vi "Process.vi"(8 "error in":errorcluster, 11 "Inst.SPC":refnum<class "Inst.SPC.lvclass">) -> (0 "error out":errorcluster, 3 "Inst.SPC out":refnum<class "Inst.SPC.lvclass">)   [LabVIEW 2019, in "Inst.SPC.lvclass"]
doc: "---------------------------------------------------------------\nJKI State Machine Objects™\nhttp://jki.net/state-machine-objects/\nCopyright (C) 2005-2015, JKI <info@jki.net>\nALL RIGHTS RESERVED"
uses:
  Inst.SPC.lvclass
  C:/Program Files (x86)/National Instruments/LabVIEW 2019/vi.lib/JKI/JKI SMO/SMO/SMO.lvclass
  C:/Program Files (x86)/National Instruments/LabVIEW 2019/user.lib/LevyLab/Instrument Framework/SMOs/Instrument/Instrument.lvclass
  Typedefs/PrivateEvents--Inst.SPC.MessageToProcess.ctl
  <userlib>/LevyLab/Instrument Framework/SMOs/RemoteControl/Typedefs/Message--Cluster.ctl
  <vilib>/JKI/JKI SMO/SMO/SMO.lvclass/SMO.ctl
  Inst.SPC.lvclass/Inst.SPC.ctl
  <vilib>/JKI/JKI SMO/SMO/Private/ReftoDVR--SMO.vi
  <userlib>/LevyLab/Instrument Framework/Instrument Types/VSource/Instrument.VSource.lvclass
  <vilib>/JKI/JKI SMO/SMO/SMO.lvclass
  <userlib>/LevyLab/Instrument Framework/SMOs/Instrument/Instrument.lvclass
  <userlib>/LevyLab/Instrument Framework/SMOs/RemoteControl/RemoteControl.lvclass
  C:/Program Files (x86)/National Instruments/LabVIEW 2019/user.lib/LevyLab/Instrument Framework/Instrument Types/VSource/Instrument.VSource.lvclass
  Typedefs/Inst.SPC.Configuration--Cluster.ctl
panel:
  out "Status":string
  out "State History":string
  # "Instrument.SPC"
  # "SPC"
  # "For instructions on how to use the JKI State Machine Objects, examples and video tutorials, visit:\nhttp://jki.net/state-machine-objects/\n\nJKI State Machine Objects™\nhttp://jki.net/state-machine-objects/\nCopyright (C) 2005-2015, JKI <info@jki.net>\nALL RIGHTS RESERVED"
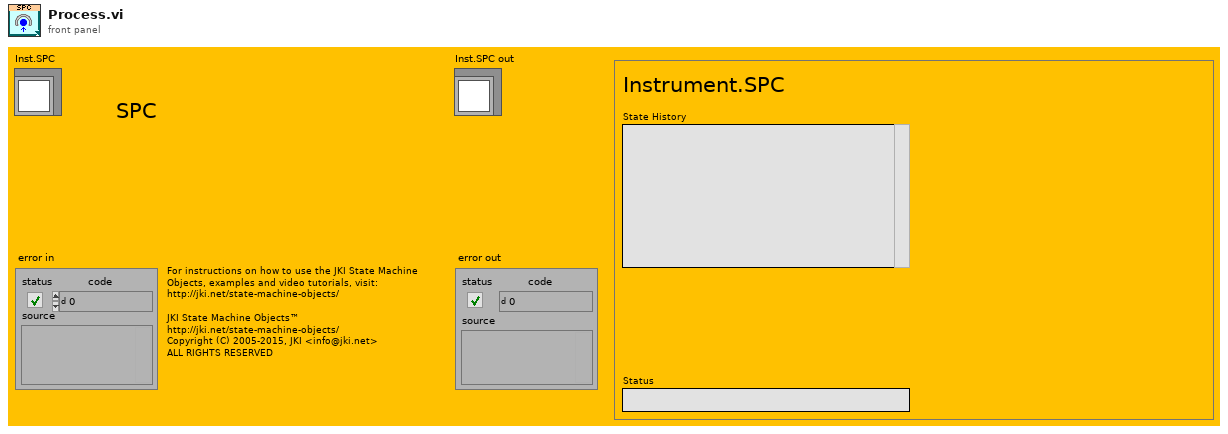
[diagram p1: front panel]
types:
  T1 = enum32{"invalid app kind", "Development System", "Run Time System", "Student Edition", "Embedded LabVIEW", "Evaluation", "Custom"}
  T2 = enum32{"Invalid", "Standard", "Closed", "Hidden", "Minimized", "Maximized"}
  T3 = typedef "Inst.SPC.lvclass/Inst.SPC.Configuration--Cluster.ctl" = cluster{"DCC_DLL":path, "SPC_DLL":path, "DCC_Serials":string[], "SPC_Serials":string[]}
  T4 = typedef "RemoteControl.lvclass/Message--Cluster.ctl" = cluster{"Command":string, "Data":variant, "ID":string}
  T5 = typedef "Inst.SPC.lvclass/PrivateEvents--Inst.SPC.MessageToProcess.ctl" = cluster{"Message":T4}
  T6 = cluster{"Core":cluster{"Current VI Reference":refnum<vi>, "Close Panel on Exit?":bool, "Last Error":cluster{"error":errorcluster, "previous state":string, "remaining states":string}, "Shutdown?":bool}, "SelfRef":refnum<class "Inst.SPC.lvclass">, "Running Step":i32, "sequence":string[], "MessageToProcess":T5}
  T7 = cluster{"Current VI Reference":refnum<vi>, "Close Panel on Exit?":bool, "Last Error":cluster{"error":errorcluster, "previous state":string, "remaining states":string}, "Shutdown?":bool}
  T8 = typedef "SMO.lvclass/Protected Events.ctl" = cluster{"StopProcesses":refnum<user-event>, "AbortProcesses":refnum<user-event>, "Config Changed":refnum<user-event>, "Dependency":refnum<user-event>}
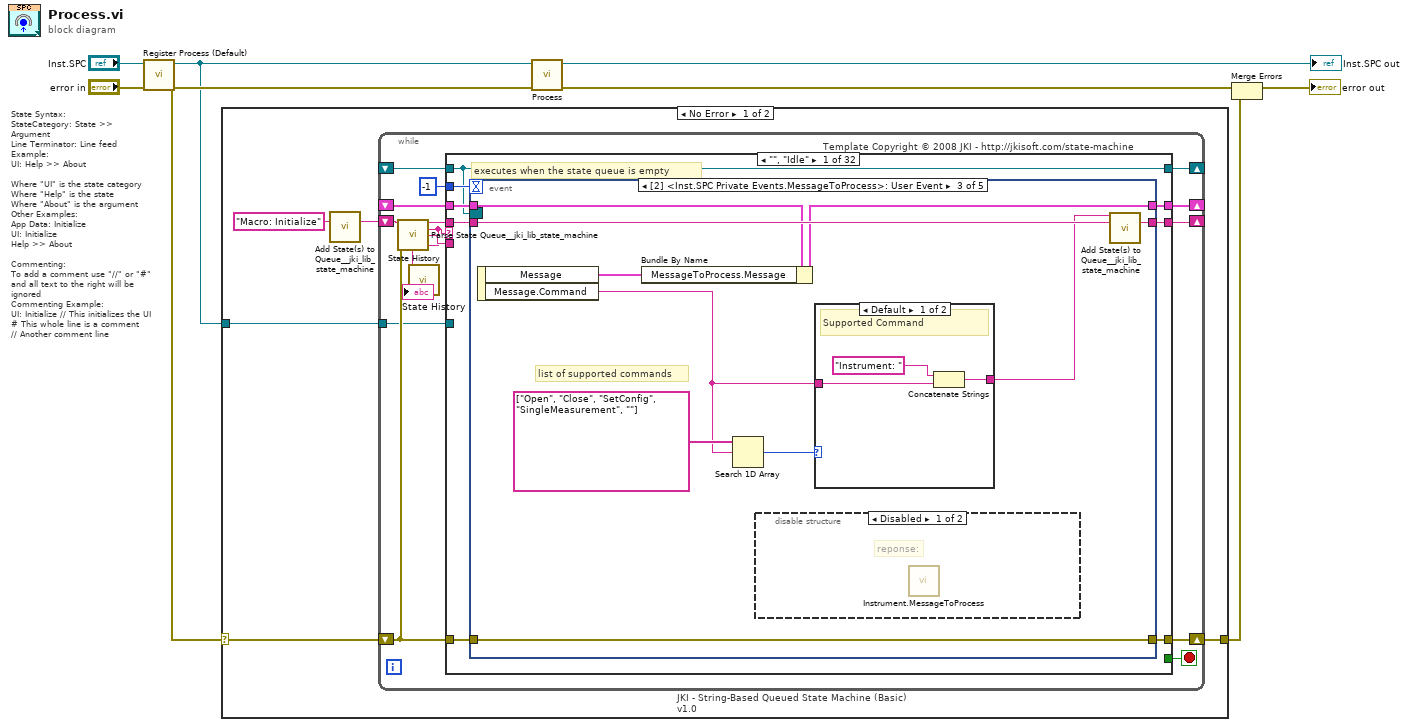
[diagram p0: block diagram]
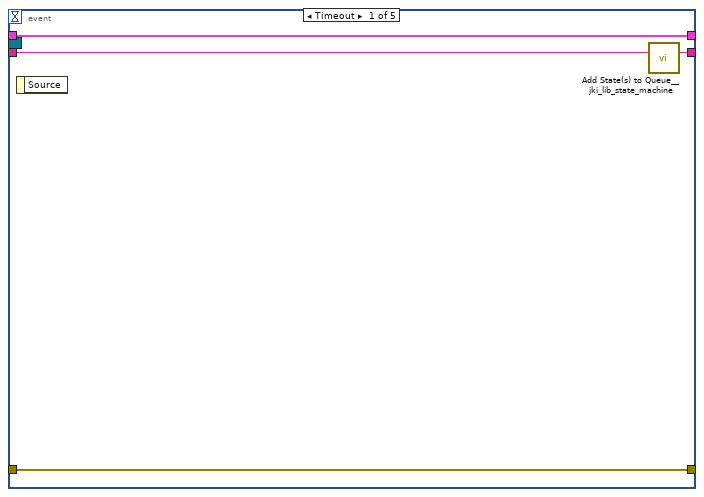
[diagram p2: hidden frame]
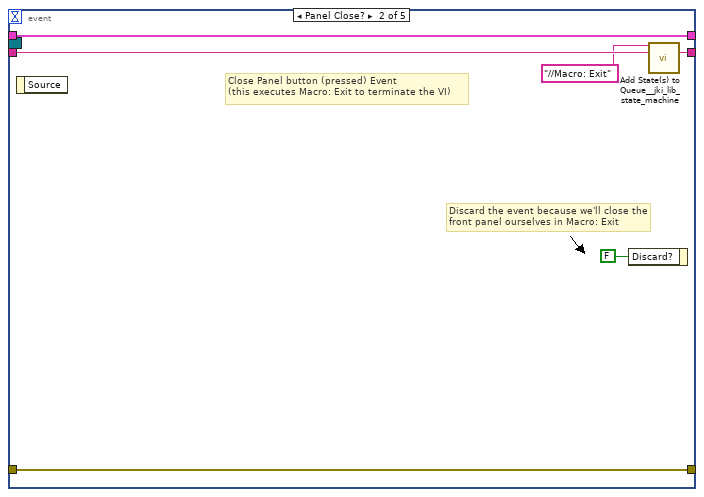
[diagram p3: hidden frame]
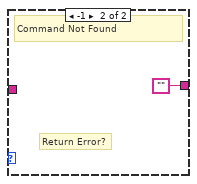
[diagram p5: hidden frame]
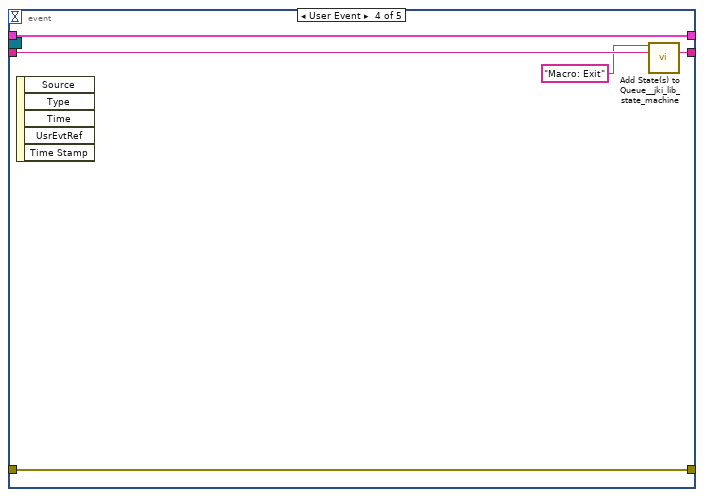
[diagram p6: hidden frame]
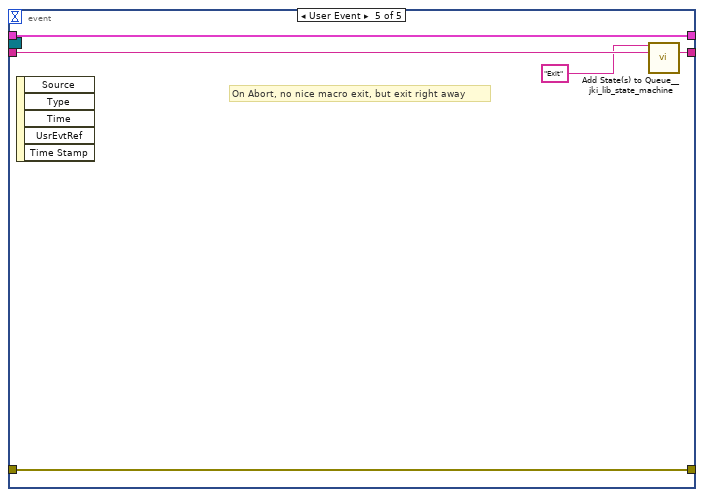
[diagram p7: hidden frame]
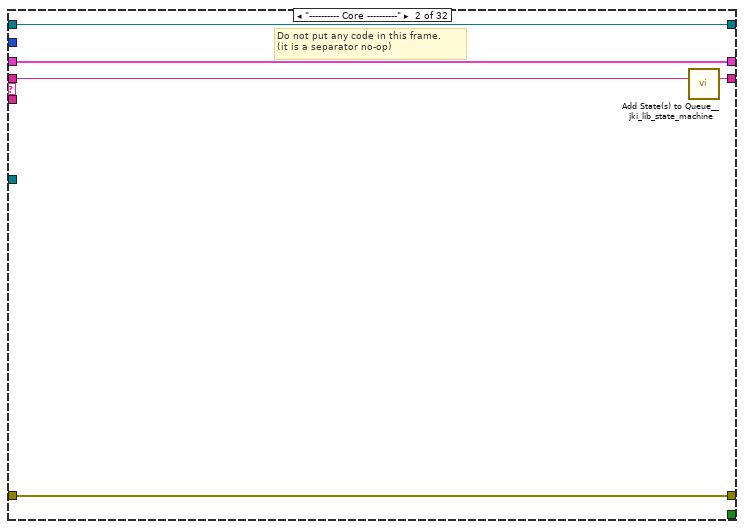
[diagram p8: hidden frame]
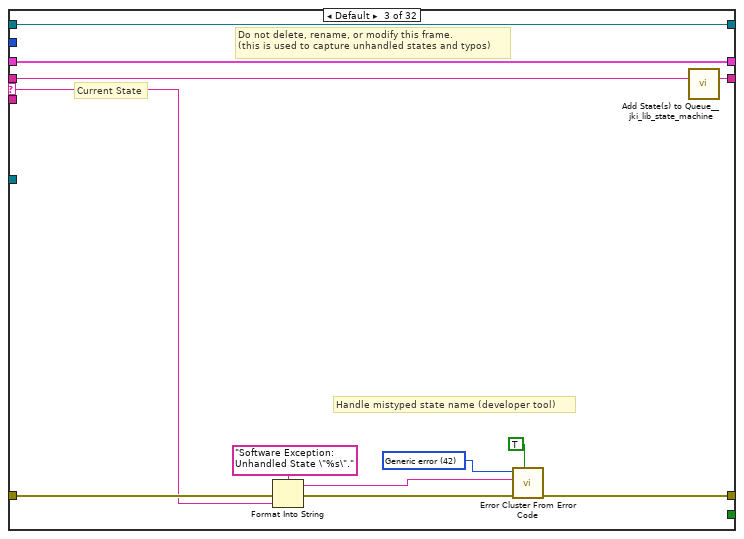
[diagram p9: hidden frame]
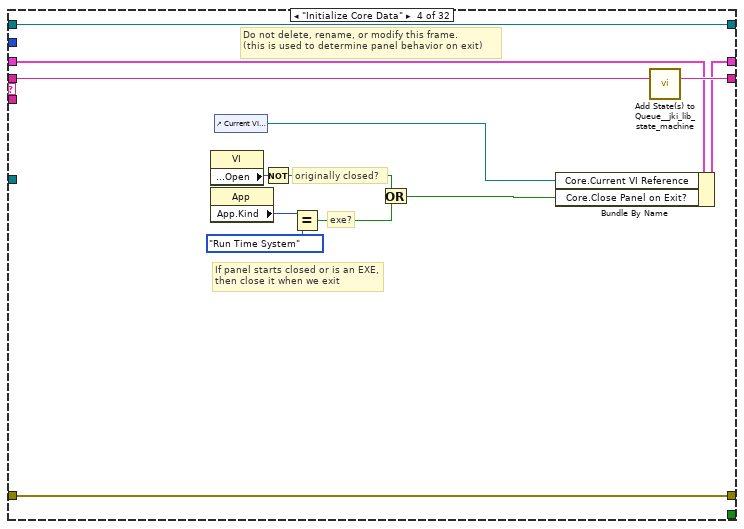
[diagram p10: hidden frame]
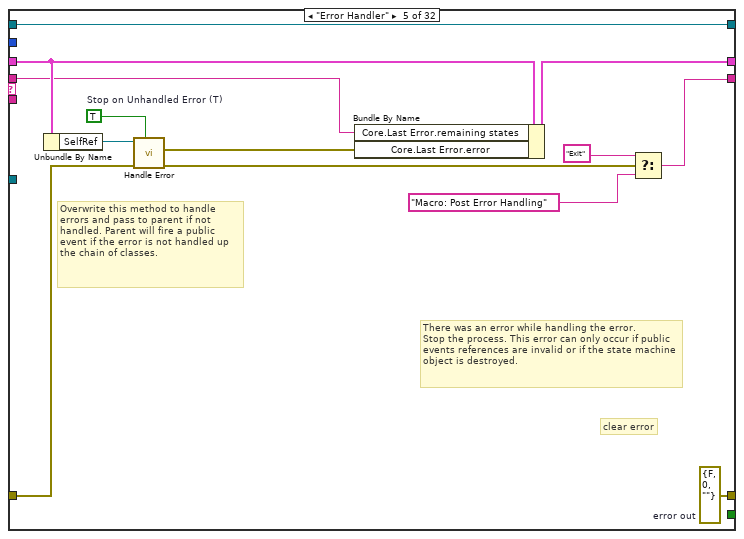
[diagram p11: hidden frame]
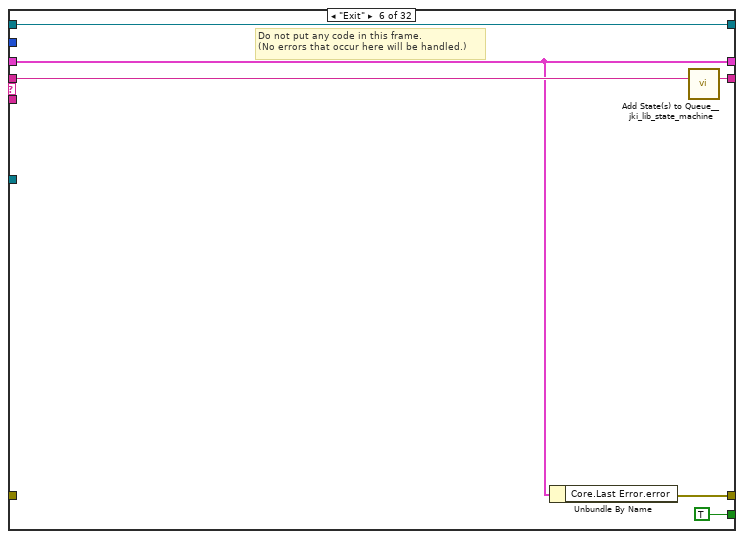
[diagram p12: hidden frame]
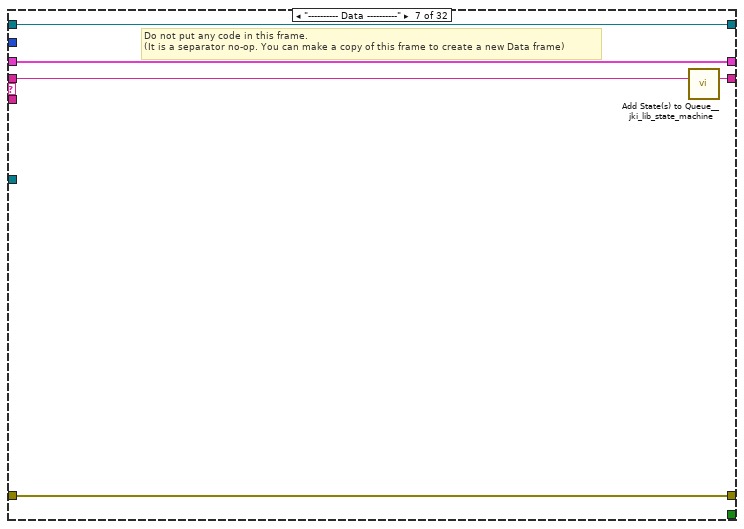
[diagram p13: hidden frame]
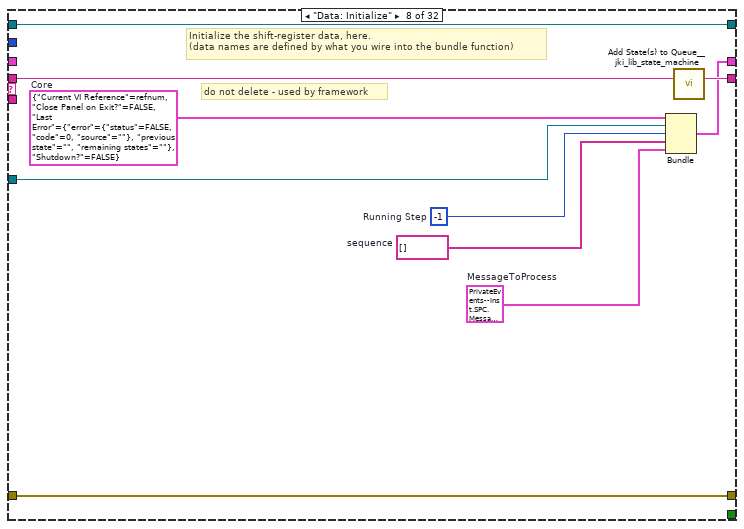
[diagram p14: hidden frame]
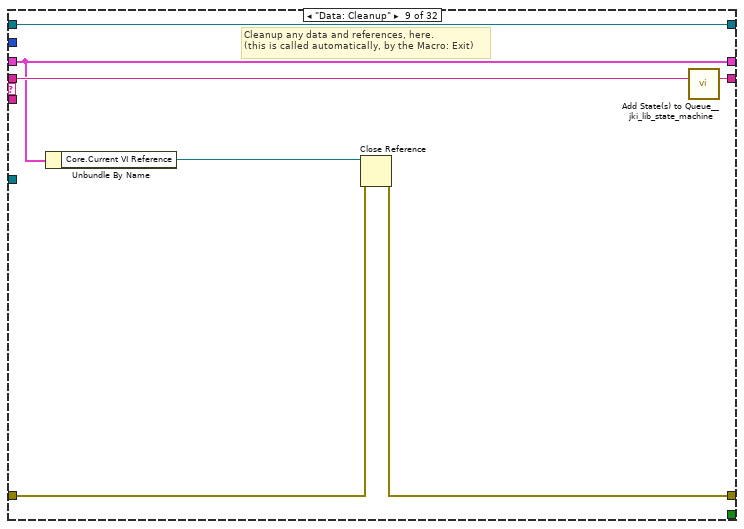
[diagram p15: hidden frame]
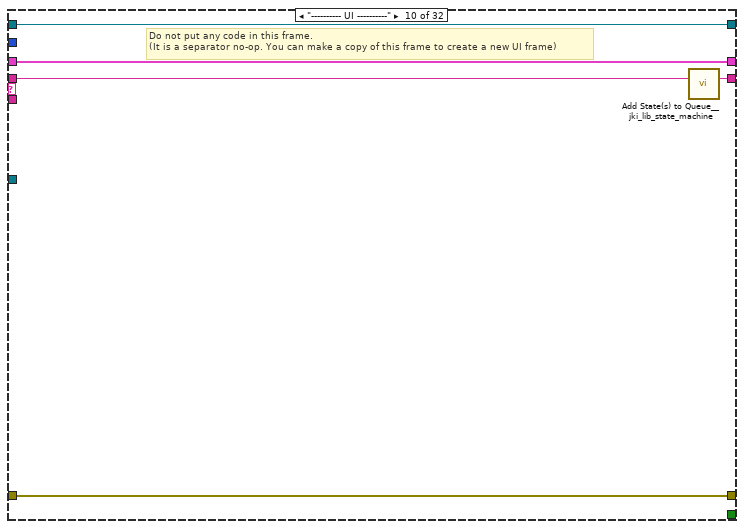
[diagram p16: hidden frame]
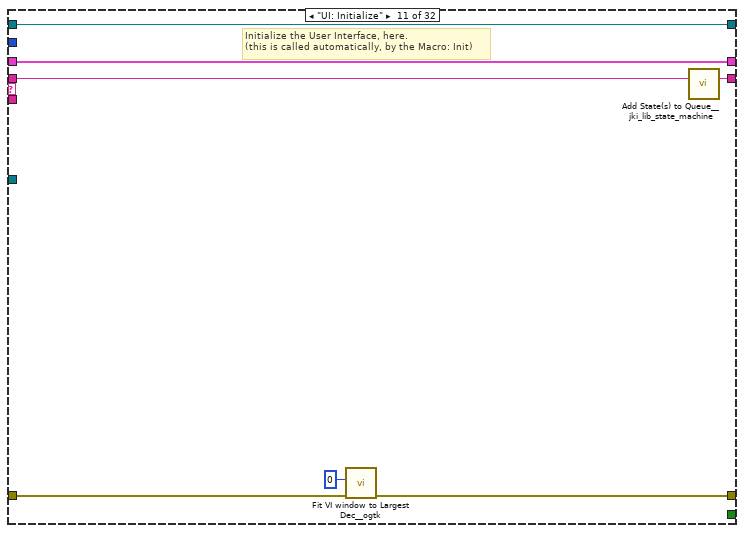
[diagram p17: hidden frame]
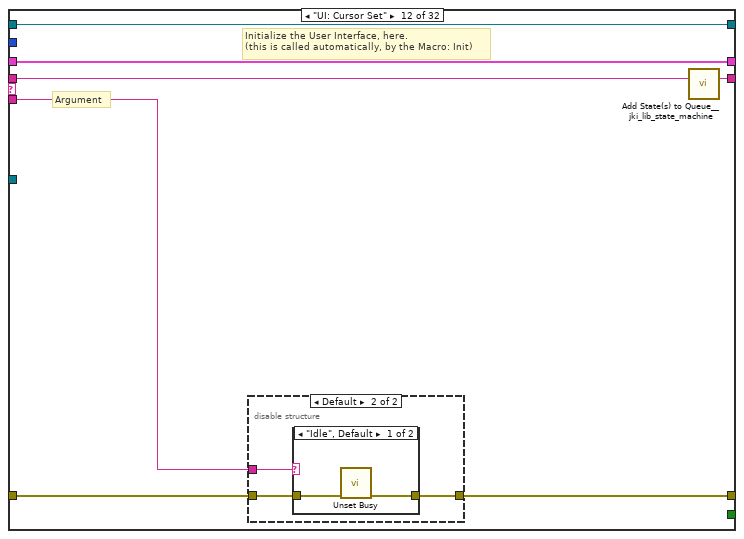
[diagram p18: hidden frame]
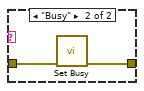
[diagram p20: hidden frame]
diagram:
  # "State Syntax:\nStateCategory: State >> Argument\nLine Terminator: Line feed\nExample:\nUI: Help >> About\n\nWhere \"UI\" is the state category\nWhere \"Help\" is the state\nWhere \"About\" is the argument\nOther Examples:\nApp Data: Initialize\nUI: Initialize\nHelp >> About\n\nCommenting:\nTo add a comment use \"//\" or \"#\" and all text to the right will be ignored\nCommenting Example:\nUI: Initialize // This initializes the UI\n# This whole line is a comment\n// Another comment line"
  n1 = call <vilib>:"Register Process (Default).vi"("error in (no error)"="error in", "SMO"="Inst.SPC") -> ("error out"=w5:errorcluster, "SelfRef"=w4:refnum<class "Inst.SPC.lvclass">)  [unwired: 8 in]
  n2 = case shown="No Error" w5 {
    selector: w5 -> [w10 w422]
    tunnel: w4 -> [w11 _]
    tunnel: [w9 w422] -> w1
    frame No Error {
      n3 = call <vilib>:"Add State(s) to Queue__jki_lib_state_machine.vi"("State(s) in (\"\")"="Macro: Initialize") -> ("States Out"=w13:string)  [unwired: 14 in]
      n4 = while "JKI - String-Based Queued State Machine (Basic) v1.0" {
        shift-right: [w22] -> _
        shift-left: _ -> [w21]
        shift-right: [w25] -> w9
        shift-left: w10 -> [w19]
        shift-right: [w24] -> _
        shift-left: w13 -> [w26]
        tunnel: w11 -> [w18]
        shift-right: [w17] -> _
        shift-left: _ -> [w16]
        stop <- w23 stop-if-true
        # "Template Copyright © 2008 JKI - http://jkisoft.com/state-machine"
        n5 = call <vilib>:"Parse State Queue__jki_lib_state_machine.vi"("State Queue"=w26, "Error In (no error)"=w19) -> ("Remaining States"=w28:string, "Current State"=w15:string, "Arguments"=w27:string)  [unwired: 11 in]
        n6 = call <userlib>:"State History.vi"("Current State"=w15) -> ("History"=→"State History":string)  [unwired: 10 in]
        n7 = case shown="\"\", \"Idle\"" w15 {
          selector: w15 -> [_ _ w77 _ _ _ _ _ _ _ _ _ _ _ _ _ _ _ _ _ _ _ _ _ _ _ _ _ _ _ _ _]
          tunnel: w28 -> [w36 w75 w81 w100 w105 w119 w124 w134 w141 w146 w153 w160 w176 w208 w227 w239 w260 w282 w287 w298 w303 w316 w322 w329 w341 w350 w357 w367 w382 w396 w402 w421]
          tunnel: w27 -> [_ _ _ _ _ _ _ _ _ _ _ w154 w170 _ _ _ _ _ _ _ _ _ _ _ _ _ _ _ _ _ w397 w405]
          tunnel: w21 -> [w34 w72 w79 w91 w109 w115 w121 _ w136 w143 w151 w158 w172 w205 w224 w229 w250 w263 w284 w295 w300 w309 w320 w324 w337 w346 w353 w363 w378 w392 w398 w411]
          tunnel: [w33 w73 w83 w97 w110 w114 w122 w126 w137 w144 w148 w155 w173 w206 w212 w237 w258 w265 w285 w289 w301 w312 w318 w326 w335 w343 w351 w361 w372 w393 w399 w413] -> w25
          tunnel: w19 -> [w32 w73 w82 w97 w111 _ w122 w126 w138 w144 w147 w156 w174 w206 w216 w237 w258 w266 w285 w290 w301 w306 w318 w326 w334 w342 w351 w361 w376 w393 w399 w407]
          tunnel: [w35 w74 w80 w99 w101 w118 w123 w133 w140 w145 w152 w159 w175 w207 w226 w238 w259 w281 w286 w297 w302 w315 w321 w328 w340 w349 w356 w366 w381 w395 w401 w420] -> w24
          tunnel: [_ _ _ _ _ TRUE _ _ _ _ _ _ _ _ _ _ _ _ _ _ _ _ _ _ _ _ _ _ _ _ _ _] -> w23
          tunnel: [w31 w72 w79 w98 w108 w115 w121 w132 w136 w143 w151 w158 w172 w205 w224 w230 w251 w263 w284 w295 w300 w309 w320 w325 w338 w347 w354 w364 w379 w392 w398 w410] -> w22
          tunnel: -1 ("Timeout") -> [w30 _ _ _ _ _ _ _ _ _ _ _ _ _ _ _ _ _ _ _ _ _ _ _ _ _ _ _ _ _ _ _]
          tunnel: w18 -> [_ _ _ _ _ _ _ w127 _ _ _ _ _ _ w220 _ _ w262 _ _ _ _ _ _ _ _ _ _ _ _ _ _]
          tunnel: [w29 w71 w76 w88 w113 w116 w120 w131 w135 w142 w150 w157 w169 w204 w225 w236 w257 w276 w283 w296 w299 w314 w319 w327 w339 w348 w355 w365 w380 w394 w400 w419] -> w17
          tunnel: w16 -> [w29 w71 w76 w88 w113 w116 w120 w131 w135 w142 w150 w157 w169 w204 w225 w236 w257 w276 w283 w296 w299 _ w319 w327 w339 w348 w355 w365 w380 w394 w400 w419]
          frame "", "Idle" {
            # "executes when the state queue is empty"
            n8 = event shown="[2] <Inst.SPC Private Events.MessageToProcess>: User Event" {
              selector: w29 -> [_ _ _ _ _]
              dyn-events: _ -> [_ _ _ _ _]
              timeout: w30 -> [_ _ _ _ _]
              tunnel: w36 -> [w40 w46 w56 w65 w70]
              tunnel: [w39 w45 w55 w64 w69] -> w35
              tunnel: w34 -> [w37 w43 w48 w62 w67]
              tunnel: [w38 w44 w54 w63 w68] -> w33
              tunnel: w32 -> [w38 w44 w54 w63 w68]
              tunnel: [w37 w43 w49 w62 w67] -> w31
              event Timeout {
                n9 = event-data() -> ()  [unwired: 1 in, 1 out]
                n10 = call <vilib>:"Add State(s) to Queue__jki_lib_state_machine.vi"("State(s) in (\"\")"=w40) -> ("States Out"=w39:string)  [unwired: 14 in]
              }
              event Panel Close? {
                # "Discard the event because we'll close the front panel ourselves in Macro: Exit"
                # "Close Panel button (pressed) Event\n(this executes Macro: Exit to terminate the VI)"
                n11 = event-data() -> ()  [unwired: 1 in, 1 out]
                n12 = event-data("Discard?"=FALSE) -> ()  [unwired: 1 in, 1 out]
                n13 = call <vilib>:"Add State(s) to Queue__jki_lib_state_machine.vi"("State(s) in Front (\"\")"="//Macro: Exit", "State(s) in (\"\")"=w46) -> ("States Out"=w45:string)  [unwired: 13 in]
              }
              event User Event {
                # "list of supported commands"
                n14 = event-data() -> ("Message"=w47:T4, "Message.Command"=w50:string)  [unwired: 1 in]
                n15 = Bundle By Name(cluster=w48, "MessageToProcess.Message"=w47) -> (w49:T6)
                n16 = Search 1D Array(1D array=string[] ["Open", "Close", "SetConfig", "SingleMeasurement", ""], element=w50) -> (index of element=w53:i32)  [unwired: 1 in]
                n17 = disable-structure shown="Disabled" {
                  frame Disabled {
                    # "reponse:"
                    n18 = call <userlib>:"Instrument.MessageToProcess.vi"() -> ()  [unwired: 10 in, 2 out]
                  }
                  frame Enabled {
                  }
                }
                n19 = case shown="Default" w53 {
                  tunnel: [w59 "" ("Empty String Constant")] -> w51
                  tunnel: w50 -> [w58 _]
                  frame Default {
                    # "Supported Command"
                    n20 = Concatenate Strings("Instrument: ", w58) -> (w59:string)
                  }
                  frame -1 {
                    # "Return Error?"
                    # "Command Not Found"
                  }
                }
                n21 = call <vilib>:"Add State(s) to Queue__jki_lib_state_machine.vi"("State(s) in Front (\"\")"=w51, "State(s) in (\"\")"=w56) -> ("States Out"=w55:string)  [unwired: 13 in]
              }
              event User Event {
                n22 = event-data() -> ()  [unwired: 1 in, 5 out]
                n23 = call <vilib>:"Add State(s) to Queue__jki_lib_state_machine.vi"("State(s) in Front (\"\")"="Macro: Exit", "State(s) in (\"\")"=w65) -> ("States Out"=w64:string)  [unwired: 13 in]
              }
              event User Event {
                # "On Abort, no nice macro exit, but exit right away"
                n24 = event-data() -> ()  [unwired: 1 in, 5 out]
                n25 = call <vilib>:"Add State(s) to Queue__jki_lib_state_machine.vi"("State(s) in Front (\"\")"="Exit", "State(s) in (\"\")"=w70) -> ("States Out"=w69:string)  [unwired: 13 in]
              }
            }
          }
          frame "---------- Core ----------" {
            # "Do not put any code in this frame.\n(it is a separator no-op)"
            n26 = call <vilib>:"Add State(s) to Queue__jki_lib_state_machine.vi"("State(s) in (\"\")"=w75) -> ("States Out"=w74:string)  [unwired: 14 in]
          }
          frame Default {
            w86 = 42 items=["No error", "Argument error", "Memory is full", "Out of zone", "End of file", "File already open", "Generic file I/O error", "File not found", "File permission error", "Disk is full", "Duplicate path", "Too many files open", "System feature not enabled", "Resource file not found", "Cannot add resource", "Resource not found", "Image not found", "Image memory error", "Pen does not exist", "Config type invalid", "Config token not found", "Config parse error", "Config memory error", "Bad external code format", "Bad external code offset", "External code not present", "Null window", "Destroy window error", "Null menu", "Print aborted", "Bad print record", "Print driver error", "Windows error during printing", "Memory error during printing", "Print dialog error", "Generic print error", "Invalid device refnum", "Device not found", "Device parameter error", "Device unit error", "Cannot open device", "Device call aborted", "Generic error", "Cancelled by user", "Object ID too low", "Object ID too high", "Object not in heap", "Unknown heap", "Unknown object (invalid DefProc)", "Unknown object (DefProc not in table)", "Message out of range", "Invalid (null) method", "Unknown message", "Manager call not supported", "Bad address", "Network operation in progress", "Network operation timed out", "Connection is busy", "Network attribute not supported", "Network error", "Address in use", "System out of memory", "Connection aborted", "Connection refused", "Not connected", "Already connected", "Connection closed", "Initialization error (interapplication manager)", "Bad occurrence", "Wait on unbound occurrence handler", "Occurrence queue overflow", "Datalog type conflict", "Unused", "Unrecognized type (interapplication manager)", "Memory corrupt", "Failed to make temporary DLL", "Old CIN version", "Drag socket not found", "Failed to load drop-object", "Failed to register OLE object", "Failed to release OLE object", "Format specifier type mismatch", "Unknown format specifier", "Too few format specifiers", "Too many format specifiers", "Scan failed", "Newer CIN version", "Error converting to variant", "Runtime menu error", "Password tampered", "Variant attribute not found", "Incompatible variant data type", "Event data is not available", "Event Store is not present", "Occurrence is not found", "Event Queue is not created", "Event info is not available", "Refnum passed is NULL", "Error retrieving Class GUID", "Error retrieving CoClass GUID", "Error retrieving TypeLib GUID.", "Bad built application magic bytes.", "Specific driver is different from the specific driver associated with the Logical Name.", "There is no session opened to the class driver.", "Max Error", "MAX - Error with config objects", "MAX - Error loading configuration", "MAX - Group not supported"]
            # "Current State"
            # "Do not delete, rename, or modify this frame.\n(this is used to capture unhandled states and typos)"
            # "Handle mistyped state name (developer tool)"
            n27 = Format Into String(format string="Software Exception: Unhandled State \"%s\"." ("message"), error in=w82, w77) -> (resulting string=w85:string, error out=w84:errorcluster)  [unwired: 1 in]
            n28 = call <vilib>:"Error Cluster From Error Code.vi"("show call chain? (False)"=TRUE, "error in (no error)"=w84, "error message (\"\")"=w85, "error code (0)"=w86) -> ("error out"=w83:errorcluster)  [unwired: 5 in]
            n29 = call <vilib>:"Add State(s) to Queue__jki_lib_state_machine.vi"("State(s) in (\"\")"=w81) -> ("States Out"=w80:string)  [unwired: 14 in]
          }
          frame "Initialize Core Data" {
            # "Do not delete, rename, or modify this frame.\n(this is used to determine panel behavior on exit)"
            # "originally closed?"
            # "exe?"
            # "If panel starts closed or is an EXE, then close it when we exit"
            n30 = property class="VI"() -> ("Front Panel.Open"=w96:bool)  [unwired: 2 in, 2 out]
            n31 = property class="App"() -> ("App.Kind"=w95:T1)  [unwired: 2 in, 2 out]
            n32 = control-ref of="Current VI Reference"() -> (w89:refnum<vi>)
            n33 = Not(x=w96) -> (.not. x?=w93:bool)
            n34 = Equal?(x=w95, y=T1."Run Time System" ("Application:Kind")) -> (x = y?=w92:bool)
            n35 = Or(x=w93, y=w92) -> (x .or. y?=w90:bool)
            n36 = Bundle By Name(cluster=w91, "Core.Current VI Reference"=w89, "Core.Close Panel on Exit?"=w90) -> (w98:T6)
            n37 = call <vilib>:"Add State(s) to Queue__jki_lib_state_machine.vi"("State(s) in (\"\")"=w100) -> ("States Out"=w99:string)  [unwired: 14 in]
          }
          frame "Error Handler" {
            w106 = TRUE  # Stop on Unhandled Error (T)
            w110 = errorcluster {"status"=FALSE, "code"=0, "source"=""}  # error out
            # "clear error"
            # "There was an error while handling the error.\nStop the process. This error can only occur if public events references are invalid or if the state machine object is destroyed."
            # "Overwrite this method to handle errors and pass to parent if not handled. Parent will fire a public event if the error is not handled up the chain of classes."
            n38 = Unbundle By Name(w109) -> ("SelfRef"=w112:refnum<class "Inst.SPC.lvclass">)
            n39 = call-dynamic "Handle Error.vi"("Stop on Unhandled Error (T)"=w106, "error in"=w111, "SMO"=w112) -> ("handling error"=w102:errorcluster, "Unhandled error"=w107:errorcluster)  [unwired: 6 in, 1 out]
            n40 = Bundle By Name(cluster=w109, "Core.Last Error.remaining states"=w105, "Core.Last Error.error"=w107) -> (w108:T6)
            n41 = Select(t="Exit", s=w102, f="Macro: Post Error Handling") -> (s? t:f=w101:string)
          }
          frame "Exit" {
            # "Do not put any code in this frame.\n(No errors that occur here will be handled.)"
            n42 = Unbundle By Name(w115) -> ("Core.Last Error.error"=w114:errorcluster)
            n43 = call <vilib>:"Add State(s) to Queue__jki_lib_state_machine.vi"("State(s) in (\"\")"=w119) -> ("States Out"=w118:string)  [unwired: 14 in]
          }
          frame "---------- Data ----------" {
            # "Do not put any code in this frame.\n(It is a separator no-op. You can make a copy of this frame to create a new Data frame)"
            n44 = call <vilib>:"Add State(s) to Queue__jki_lib_state_machine.vi"("State(s) in (\"\")"=w124) -> ("States Out"=w123:string)  [unwired: 14 in]
          }
          frame "Data: Initialize" {
            w125 = T5 {"Message"={"Command"="", "Data"=variant(string ""), "ID"=""}}  # MessageToProcess
            w128 = string[] []  # sequence
            w129 = -1  # Running Step
            w130 = T7 {"Current VI Reference"=refnum, "Close Panel on Exit?"=FALSE, "Last Error"={"error"={"status"=FALSE, "code"=0, "source"=""}, "previous state"="", "remaining states"=""}, "Shutdown?"=FALSE}  # Core
            # "do not delete - used by framework"
            # "Initialize the shift-register data, here.\n(data names are defined by what you wire into the bundle function)"
            n45 = Bundle("Core"=w130, "SelfRef"=w127, "Running Step"=w129, "sequence"=w128, "MessageToProcess"=w125) -> (w132:T6)  [unwired: 1 in]
            n46 = call <vilib>:"Add State(s) to Queue__jki_lib_state_machine.vi"("State(s) in (\"\")"=w134) -> ("States Out"=w133:string)  [unwired: 14 in]
          }
          frame "Data: Cleanup" {
            # "Cleanup any data and references, here.\n(this is called automatically, by the Macro: Exit)"
            n47 = Unbundle By Name(w136) -> ("Core.Current VI Reference"=w139:refnum<vi>)
            n48 = Close Reference(reference=w139, error in (no error)=w138) -> (error out=w137:errorcluster)
            n49 = call <vilib>:"Add State(s) to Queue__jki_lib_state_machine.vi"("State(s) in (\"\")"=w141) -> ("States Out"=w140:string)  [unwired: 14 in]
          }
          frame "---------- UI ----------" {
            # "Do not put any code in this frame.\n(It is a separator no-op. You can make a copy of this frame to create a new UI frame)"
            n50 = call <vilib>:"Add State(s) to Queue__jki_lib_state_machine.vi"("State(s) in (\"\")"=w146) -> ("States Out"=w145:string)  [unwired: 14 in]
          }
          frame "UI: Initialize" {
            # "Initialize the User Interface, here.\n(this is called automatically, by the Macro: Init)"
            n51 = call <userlib>:"Fit VI window to Largest Dec__ogtk.vi"("error in (no error)"=w147, "border spacing (2 px)"=0) -> ("error out"=w148:errorcluster)  [unwired: 4 in, 1 out]
            n52 = call <vilib>:"Add State(s) to Queue__jki_lib_state_machine.vi"("State(s) in (\"\")"=w153) -> ("States Out"=w152:string)  [unwired: 14 in]
          }
          frame "UI: Cursor Set" {
            # "Argument"
            # "Initialize the User Interface, here.\n(this is called automatically, by the Macro: Init)"
            n53 = disable-structure shown="Default" {
              disable-tunnel: w156 -> [w161 w164]
              disable-tunnel: [w161 w163] -> w155
              disable-tunnel: w154 -> [_ w162]
              frame condition #0 {
              }
              frame condition #1 (active) {
                n54 = case shown="\"Idle\", Default" w162 {
                  tunnel: w164 -> [w166 w168]
                  tunnel: [w165 w167] -> w163
                  frame "Idle", Default {
                    n55 = call <vilib>:"Unset Busy.vi"("error in (no error)"=w166) -> ("error out"=w165:errorcluster)  [unwired: 10 in]
                  }
                  frame "Busy" {
                    n56 = call <vilib>:"Set Busy.vi"("error in (no error)"=w168) -> ("error out"=w167:errorcluster)  [unwired: 9 in, 1 out]
                  }
                }
              }
            }
            n57 = call <vilib>:"Add State(s) to Queue__jki_lib_state_machine.vi"("State(s) in (\"\")"=w160) -> ("States Out"=w159:string)  [unwired: 14 in]
          }
          frame "UI: Front Panel State" {
            # "Argument"
            # "Set Front Panel Open or Closed\n(Usage: \"UI: Front Panel State >> Open|Close\")"
            n58 = Unbundle By Name(w172) -> ("Core.Current VI Reference"=w171:refnum<vi>)
            n59 = disable-structure shown="TARGET_TYPE==RT" {
              disable-tunnel: w174 -> [w180 w203]
              disable-tunnel: [w179 w203] -> w173
              disable-tunnel: w171 -> [w178 _]
              disable-tunnel: w170 -> [w177 _]
              frame condition #0 (active) {
                n60 = case shown="\"Close\"" w177 {
                  tunnel: w180 -> [w184 w197]
                  tunnel: [w186 w198] -> w179
                  tunnel: w178 -> [w185 w195]
                  frame "Open", Default {
                    n61 = property class="VI"(reference=w185, error in=w184) -> (reference out=w182:refnum<vi>, error out=w183:errorcluster, "FP.State"=w181:T2)
                    n62 = case shown="\"Closed\"" w181 {
                      tunnel: [w189 w192] -> w186
                      tunnel: w183 -> [w188 w192]
                      tunnel: w182 -> [w187 _]
                      frame "Closed" {
                        n63 = invoke class="VI" method="FP.Open"(reference=w187, error in=w188, "Activate"=TRUE, "State"=T2."Standard") -> (error out=w189:errorcluster)  [unwired: 1 in, 4 out]
                      }
                      frame Default {
                      }
                    }
                  }
                  frame "Close" {
                    n64 = property class="VI"(reference=w195, error in=w197) -> (reference out=w194:refnum<vi>, error out=w196:errorcluster, "FP.State"=w193:T2)
                    n65 = case shown="Default" w193 {
                      tunnel: [w199 w202] -> w198
                      tunnel: w196 -> [w199 w201]
                      tunnel: w194 -> [_ w200]
                      frame "Invalid", "Closed" {
                      }
                      frame Default {
                        n66 = invoke class="VI" method="FP.Close"(reference=w200, error in=w201) -> (error out=w202:errorcluster)  [unwired: 1 in, 2 out]
                      }
                    }
                  }
                }
              }
              frame condition #1 {
              }
            }
            n67 = call <vilib>:"Add State(s) to Queue__jki_lib_state_machine.vi"("State(s) in (\"\")"=w176) -> ("States Out"=w175:string)  [unwired: 14 in]
          }
          frame "---------- Macro ----------" {
            # "Do not put any code in this frame.\n(It is a separator no-op. You can make a copy of this frame to create a new Macro frame)"
            n68 = call <vilib>:"Add State(s) to Queue__jki_lib_state_machine.vi"("State(s) in (\"\")"=w208) -> ("States Out"=w207:string)  [unwired: 14 in]
          }
          frame "Macro: Initialize" {
            # "Initialization Macro\n(This is called once, when the VI starts)"
            n69 = call-dynamic "Read Debug Mode.vi"("error in (no error)"=w216, "Instrument in"=w220) -> ("error out"=w215:errorcluster, "Debug Mode?"=w217:bool)  [unwired: 7 in, 1 out]
            n70 = call <userlib>:"Wait (ms)__ogtk.vi"("error in (no error)"=w215, "milliseconds to wait"=u32 0) -> ("error out"=w212:errorcluster)  [unwired: 8 in, 1 out]
            n71 = Select(t="Open", s=w217, f="Close") -> (s? t:f=w213:string)
            n72 = Format Into String(format string="UI: Initialize\nUI: Front Panel State >> %s\nInstrument: Open Hardware", initial string="", w213) -> (resulting string=w214:string)  [unwired: 1 in, 1 out]
            n73 = call <vilib>:"Add State(s) to Queue__jki_lib_state_machine.vi"("State(s) in Front (\"\")"="Data: Initialize\nInitialize Core Data\nEvents: Register", "State(s) in (\"\")"="Process: Sync", "State(s) at Back (\"\")"=w214) -> ("States Out"=w222:string)  [unwired: 12 in]
            n74 = call <vilib>:"Add State(s) to Queue__jki_lib_state_machine.vi"("State(s) in Front (\"\")"=w222, "State(s) in (\"\")"=w227) -> ("States Out"=w226:string)  [unwired: 13 in]
          }
          frame "Macro: Post Error Handling" {
            # "Clear Last Error?"
            n75 = Unbundle By Name(w229) -> ("Core.Last Error.remaining states"=w231:string, "Core.Shutdown?"=w232:bool)
            n76 = Unbundle By Name(w229) -> ("Core.Last Error.error"=w235:errorcluster)
            n77 = case shown="False" FALSE {
              tunnel: w235 -> [w243 _]
              tunnel: [w243 _] -> w234
              frame False {
              }
              frame True {
              }
            }
            n78 = case shown="True" w232 {
              tunnel: w231 -> [w240 w242]
              tunnel: [w240 w241] -> w228
              frame False {
                # "These are the remaining states (at the moment the error occured). States can be altered according to business logic."
                # "NOT SHUTTING DOWN"
              }
              frame True {
                # "Developer can decide to alter the states but should be aware that during the shutdown process, there are certain states that must be run for the SMO to properly shut itself (and this process) down. As such, one can add states to perform additional clean-ups, but should append the remaining state to be executed."
                # "SHUTTING DOWN"
                n79 = call <vilib>:"Add State(s) to Queue__jki_lib_state_machine.vi"("State(s) in (\"\")"=w242) -> ("States Out"=w241:string)  [unwired: 14 in]
              }
            }
            n80 = Bundle By Name(cluster=w229, "Core.Last Error.error"=w234) -> (w230:T6)
            n81 = call <vilib>:"Add State(s) to Queue__jki_lib_state_machine.vi"("State(s) in Front (\"\")"=w228, "State(s) in (\"\")"=w239) -> ("States Out"=w238:string)  [unwired: 13 in]
          }
          frame "Macro: Run Sequence" {
            # "0,1,2,3,4,"
            # "5"
            # "Do not put any code in this frame.\n(It is a separator no-op. You can make a copy of this frame to create a new Macro frame)"
            n82 = Unbundle By Name(w250) -> ("sequence"=w246:string[], "Running Step"=w244:i32)
            n83 = Array Size(array=w246) -> (size(s)=w256:i32)
            n84 = Index Array(array=w246, index=w244) -> (element=w245:string)
            n85 = Greater Or Equal?(x=w256, y=w244) -> (x >= y?=w248:bool)
            n86 = Select(t=-1 ("Running Step"), s=w248, f=w244) -> (s? t:f=w255:i32)
            n87 = Bundle By Name(cluster=w250, "Running Step"=w255) -> (w251:T6)
            n88 = Select(t="Sequence: Status >> ...", s=w248, f="Idle //Check Event Structure\nMacro: Run Sequence" ("State(s) at Back (\"\")")) -> (s? t:f=w247:string)
            n89 = call <vilib>:"Add State(s) to Queue__jki_lib_state_machine.vi"("State(s) in Front (\"\")"=w245, "State(s) at Back (\"\")"=w247) -> ("States Out"=w249:string)  [unwired: 13 in]
            n90 = call <vilib>:"Add State(s) to Queue__jki_lib_state_machine.vi"("State(s) in Front (\"\")"=w249, "State(s) in (\"\")"=w260) -> ("States Out"=w259:string)  [unwired: 13 in]
          }
          frame "Macro: Exit" {
            # "Exit Macro\n(This is called once, when the VI exits)"
            n91 = Unbundle By Name(w263) -> ("Core.Close Panel on Exit?"=w280:bool)
            n92 = call-dynamic "Read Debug Mode.vi"("error in (no error)"=w266, "Instrument in"=w262) -> ("error out"=w265:errorcluster, "Debug Mode?"=w264:bool)  [unwired: 7 in, 1 out]
            n93 = Select(t="Open", s=w264, f="Close") -> (s? t:f=w270:string)
            n94 = call <vilib>:"Build State String with Arguments__JKI_lib_State_Machine.vi"("Arguments (\"\")"=w270, "State"="UI: Front Panel State") -> ("State with Arguments"=w267:string)  [unwired: 4 in]
            n95 = Select(t=w267, s=w280, f="" ("Empty String Constant")) -> (s? t:f=w278:string)
            n96 = call <vilib>:"Add State(s) to Queue__jki_lib_state_machine.vi"("State(s) in Front (\"\")"="Data: Cleanup\nEvents: Unregister", "State(s) in (\"\")"="Process: Sync", "State(s) at Back (\"\")"="Exit") -> ("States Out"=w273:string)  [unwired: 12 in]
            n97 = call <vilib>:"Add State(s) to Queue__jki_lib_state_machine.vi"("State(s) in Front (\"\")"="Instrument: Close Hardware", "State(s) in (\"\")"=w278, "State(s) at Back (\"\")"=w273) -> ("States Out"=w277:string)  [unwired: 12 in]
            n98 = call <vilib>:"Add State(s) to Queue__jki_lib_state_machine.vi"("State(s) in Front (\"\")"=w277, "State(s) in (\"\")"=w282) -> ("States Out"=w281:string)  [unwired: 13 in]
          }
          frame "---------- Process ----------" {
            # "Template Separator\n(You can make a copy of, or modify, this frame)"
            n99 = call <vilib>:"Add State(s) to Queue__jki_lib_state_machine.vi"("State(s) in (\"\")"=w287) -> ("States Out"=w286:string)  [unwired: 14 in]
          }
          frame "Process: Sync" {
            n100 = Unbundle By Name(w295) -> ("SelfRef"=w291:refnum<class "Inst.SPC.lvclass">)
            n101 = call <vilib>:"WaitOnProcessSync.vi"("error in (no error)"=w290, "SMO"=w291) -> ("error out"=w289:errorcluster, "Don't run?"=w294:bool)  [unwired: 7 in, 1 out]
            n102 = Select(t="Data: Cleanup\nEvents: Unregister\nExit", s=w294, f="" ("Empty String Constant")) -> (s? t:f=w288:string)
            n103 = call <vilib>:"Add State(s) to Queue__jki_lib_state_machine.vi"("State(s) in Front (\"\")"=w288, "State(s) in (\"\")"=w298) -> ("States Out"=w297:string)  [unwired: 13 in]
          }
          frame "---------- Events ----------" {
            # "Template Separator\n(You can make a copy of, or modify, this frame)"
            n104 = call <vilib>:"Add State(s) to Queue__jki_lib_state_machine.vi"("State(s) in (\"\")"=w303) -> ("States Out"=w302:string)  [unwired: 14 in]
          }
          frame "Events: Register" {
            n105 = Unbundle By Name(w309) -> ("SelfRef"=w310:refnum<class "Inst.SPC.lvclass">)
            n106 = call <vilib>:"GetProtectedEvents.vi"("SMO"=w310) -> ("error out"=w308:errorcluster, "SMO Protected Events"=w313:T8, "SMO out"=w307:refnum<class "Inst.SPC.lvclass">)  [unwired: 8 in]
            n107 = call "Inst.SPC.GetPrivateEvents.vi"("Inst.SPC in"=w307) -> ("error out"=w304:errorcluster, "Inst.SPC Private Events"=w305:cluster{"MessageToProcess":refnum<user-event>})  [unwired: 8 in, 1 out]
            n108 = register-events(w313, w305) -> (reference out=w314:refnum<event-registration>, error out=w311:errorcluster)  [unwired: 2 in]
            n109 = Merge Errors(w311, w304, w308, w306) -> (w312:errorcluster)
            n110 = call <vilib>:"Add State(s) to Queue__jki_lib_state_machine.vi"("State(s) in (\"\")"=w316) -> ("States Out"=w315:string)  [unwired: 14 in]
          }
          frame "Events: Unregister" {
            n111 = Unregister For Events(event registration refnum=w319, error in=w318) -> (error out=w317:errorcluster)
            n112 = call <vilib>:"Clear Errors.vi"("error in (no error)"=w317) -> ()  [unwired: 5 in, 2 out]
            n113 = call <vilib>:"Add State(s) to Queue__jki_lib_state_machine.vi"("State(s) in (\"\")"=w322) -> ("States Out"=w321:string)  [unwired: 14 in]
          }
          frame "---------- Instrument ----------" {
            n114 = Unbundle By Name(w324) -> ("SelfRef"=w323:refnum<class "Inst.SPC.lvclass">)
            n115 = Bundle By Name(cluster=w324, "SelfRef"=w323) -> (w325:T6)
            n116 = call <vilib>:"Add State(s) to Queue__jki_lib_state_machine.vi"("State(s) in (\"\")"=w329) -> ("States Out"=w328:string)  [unwired: 14 in]
          }
          frame "Instrument: Open Hardware" {
            # "This will call the Handle command \"SetConfig\" \nInput data from here to the Handle command which\nwill be parsed to the instrument wire."
            n117 = Unbundle By Name(w337) -> ("SelfRef"=w336:refnum<class "Inst.SPC.lvclass">)
            n118 = call-dynamic "Open Hardware.vi"("error in (no error)"=w334, "Inst.SPC in"=w336) -> ("error out"=w335:errorcluster, "Inst.SPC out"=w332:refnum<class "Inst.SPC.lvclass">)  [unwired: 8 in]
            n119 = Unbundle By Name(w332) -> ("Configuration"=w331:T3)
            n120 = call <userlib>:"Instrument.MessageToProcess.vi"("Data"=w331, "Command"="SetConfig", "Instrument"=w332) -> ("Instrument out"=w333:refnum<class "Inst.SPC.lvclass">)  [unwired: 7 in, 1 out]
            n121 = Bundle By Name(cluster=w337, "SelfRef"=w333) -> (w338:T6)
            n122 = call <vilib>:"Add State(s) to Queue__jki_lib_state_machine.vi"("State(s) in (\"\")"=w341) -> ("States Out"=w340:string)  [unwired: 14 in]
          }
          frame "Instrument: Close Hardware" {
            n123 = Unbundle By Name(w346) -> ("SelfRef"=w345:refnum<class "Inst.SPC.lvclass">)
            n124 = call-dynamic "Close Hardware.vi"("error in (no error)"=w342, "Inst.SPC in"=w345) -> ("error out"=w343:errorcluster, "Inst.SPC out"=w344:refnum<class "Inst.SPC.lvclass">)  [unwired: 8 in]
            n125 = Bundle By Name(cluster=w346, "SelfRef"=w344) -> (w347:T6)
            n126 = call <vilib>:"Add State(s) to Queue__jki_lib_state_machine.vi"("State(s) in (\"\")"=w350) -> ("States Out"=w349:string)  [unwired: 14 in]
          }
          frame "Instrument: SingleMeasurement" {
            n127 = Unbundle By Name(w353) -> ("SelfRef"=w352:refnum<class "Inst.SPC.lvclass">)
            n128 = flat-sequence {
              frame #0 {
                (unwired) u16[][] [] ("Data")
                # "SPC_start_measurement.vi....etc"
              }
            }
            n129 = Bundle By Name(cluster=w353, "SelfRef"=w352) -> (w354:T6)
            n130 = call <vilib>:"Add State(s) to Queue__jki_lib_state_machine.vi"("State(s) in (\"\")"=w357) -> ("States Out"=w356:string)  [unwired: 14 in]
          }
          frame "Instrument: SetConfig" {
            n131 = Unbundle By Name(w363) -> ("SelfRef"=w362:refnum<class "Inst.SPC.lvclass">, "MessageToProcess.Message.Data"=w360:variant)
            n132 = Variant To Data(type=T3 {"DCC_DLL"=path "", "SPC_DLL"=path "", "DCC_Serials"=["", ""], "SPC_Serials"=["", ""]} ("Configuration"), Variant=w360) -> (data=w358:T3)  [unwired: 1 in, 1 out]
            n133 = Unbundle By Name(w358) -> ()  [unwired: 1 out]
            n134 = Bundle By Name(cluster=w363, "SelfRef"=w362) -> (w364:T6)
            n135 = call <vilib>:"Add State(s) to Queue__jki_lib_state_machine.vi"("State(s) in (\"\")"=w367) -> ("States Out"=w366:string)  [unwired: 14 in]
          }
          frame "Instrument: Do Something" {
            # "communicate with\nhardware"
            n136 = Unbundle By Name(w378) -> ("SelfRef"=w377:refnum<class "Inst.SPC.lvclass">, "MessageToProcess.Message.Data"=w375:variant, "MessageToProcess.Message.ID"=w370:string)
            n137 = call "Inst.SPC.DoSomething.vi"("error in (no error)"=w376, "Data"=w375, "Inst.SPC in"=w377) -> ("error out"=w371:errorcluster, "Data out"=w369:variant, "Inst.SPC out"=w374:refnum<class "Inst.SPC.lvclass">)  [unwired: 6 in]
            n138 = Empty String/Path?(string/path=w369) -> (empty?=w368:bool)
            n139 = case shown="False" w368 {
              tunnel: w374 -> [w389 w391]
              tunnel: [w388 w391] -> w373
              tunnel: [w387 w390] -> w372
              tunnel: w369 -> [w384 _]
              tunnel: w371 -> [w383 w390]
              tunnel: w370 -> [w385 _]
              frame False {
                # "send data to\ninstrument:process.vi"
                n140 = call <userlib>:"Instrument.MessageToProcess.vi"("ID"=w385, "error in (no error)"=w383, "Data"=w384, "Command"="Set Parameter", "Instrument"=w389) -> ("error out"=w387:errorcluster, "Instrument out"=w388:refnum<class "Inst.SPC.lvclass">)  [unwired: 5 in]
              }
              frame True {
              }
            }
            n141 = Bundle By Name(cluster=w378, "SelfRef"=w373) -> (w379:T6)
            n142 = call <vilib>:"Add State(s) to Queue__jki_lib_state_machine.vi"("State(s) in (\"\")"=w382) -> ("States Out"=w381:string)  [unwired: 14 in]
          }
          frame "---------- Sequence ----------" {
            n143 = call <vilib>:"Add State(s) to Queue__jki_lib_state_machine.vi"("State(s) in (\"\")"=w396) -> ("States Out"=w395:string)  [unwired: 14 in]
          }
          frame "Sequence: Status" {
            # "Sequence: Status\n(Use this frame to pass the status to the UI, this VI's UI, etc)"
            n144 = call <vilib>:"Add State(s) to Queue__jki_lib_state_machine.vi"("State(s) in (\"\")"=w402) -> ("States Out"=w401:string)  [unwired: 14 in]
            "Status" <- w397
          }
          frame "Sequence: Wait" {
            # "Sequence: Wait\n(Non-Blocking Wait)"
            # "F = repeat this state. wait\nT = go to next state. don't wait"
            n145 = Unbundle By Name(w411) -> ("Running Step"=w404:i32)
            n146 = call <userlib>:"Wait Logic.vi"("error in (no error)"=w407, "Time"=w405) -> ("error out"=w406:errorcluster, "Status String"=w403:string, "Trigger"=w408:bool)  [unwired: 6 in, 1 out]
            n147 = Increment(x=w404) -> (x+1=w418:i32)
            n148 = Select(t=w418, s=w408, f=w404) -> (s? t:f=w409:i32)
            n149 = Select(t=u32 0, s=w408, f=u32 100 ("milliseconds to wait")) -> (s? t:f=w415:u32)
            n150 = call <userlib>:"Wait (ms)__ogtk.vi"("error in (no error)"=w406, "milliseconds to wait"=w415) -> ("error out"=w413:errorcluster)  [unwired: 8 in, 1 out]
            n151 = Bundle By Name(cluster=w411, "Running Step"=w409) -> (w410:T6)
            n152 = call <vilib>:"Build State String with Arguments__JKI_lib_State_Machine.vi"("Arguments (\"\")"=w403, "State"="Sequence: Status") -> ("State with Arguments"=w412:string)  [unwired: 4 in]
            n153 = call <vilib>:"Add State(s) to Queue__jki_lib_state_machine.vi"("State(s) in Front (\"\")"=w412, "State(s) in (\"\")"=w421) -> ("States Out"=w420:string)  [unwired: 13 in]
          }
        }
      }
    }
    frame Error {
    }
  }
  n154 = call-parent "Process.vi"("error in"=w5, "Instrument"=w4) -> ("error out"=w2:errorcluster, "Instrument out"=→"Inst.SPC out":refnum<class "Inst.SPC.lvclass">)  [unwired: 8 in]
  n155 = Merge Errors(w2, w1) -> (→"error out":errorcluster)
